vi "Arctangent_by_Quadrant.vi"(10 "Quadrature":dbl, 11 "In-Phase":dbl) -> (3 "ArcTangent":dbl)   [LabVIEW 2018]
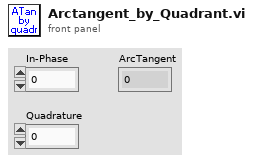
[diagram p1: front panel]
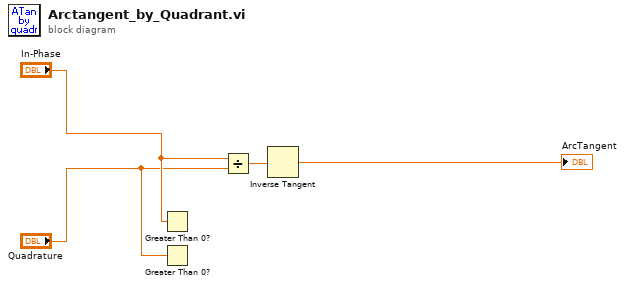
[diagram p0: block diagram]
diagram:
  n1 = Greater Than 0?(x="In-Phase") -> ()  [unwired: 1 out]
  n2 = Greater Than 0?(x="Quadrature") -> ()  [unwired: 1 out]
  n3 = Divide(x="In-Phase", y="Quadrature") -> (x/y=w3:dbl)
  n4 = Inverse Tangent(1:w3) -> (0:→"ArcTangent":dbl)
